vi "DBL to msgpack.vi"(11 "DBL":dbl) -> (3 "msgpack":u8[](array[numeric]))   [LabVIEW 2020, in "MessagePack.lvlib" / "MessagePack.lvclass"]
uses:
  MessagePack.lvclass
  Format bytes.ctl
  MessagePack.lvclass/MessagePack.ctl
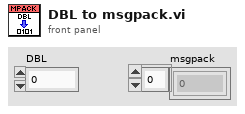
[diagram p1: front panel]
types:
  T1 = typedef "MessagePack.lvlib/MessagePack.lvclass/Format bytes.ctl" = u8
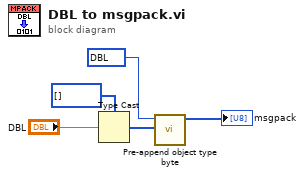
[diagram p0: block diagram]
diagram:
  w1 = T1 203 items=["nil"=192, "UINT8"=204, "UINT16"=205, "UINT32"=206, "UINT64"=207, "INT8"=208, "INT16"=209, "INT32"=210, "INT64"=211, "SGL"=202, "DBL"=203] ("Format byte")
  n1 = Type Cast(type=u8[] [] ("bytes"), x="DBL") -> (*(type *) &x=w5:u8[])
  n2 = call "Pre-append object type byte.vi"("data in"=w5, "Format byte"=w1) -> ("bytes add"=→"msgpack":u8[])  [unwired: 9 in]
